vi "DSF.Engine.Interface.Transceiver.Write.Command.vi"(6 "overwrite on timeout (T)":bool, 8 "error in (no error)":errorcluster, 9 "timeout in ms (0)":i32 format="%d ms", 10 "command":T1, 11 "Transceiver Interface in":refnum<class "DSF.Engine.Interface.Transceiver.lvclass">) -> (0 "error out":errorcluster, 1 "timed out?":bool, 3 "Transceiver Interface out":refnum<class "DSF.Engine.Interface.Transceiver.lvclass">)   [LabVIEW 2017, in "DSF.Engine.lvlib" / "DSF.Engine.Interface.Transceiver.lvclass"]
uses:
  DSF.Engine.Interface.Transceiver.lvclass
  C:/Git/DSF/Source/Engine/Classes/Interface/DSF.Engine.Interface.lvclass
  DSF.Engine.Interface.Transceiver.Command Data.ctl
  DSF.Engine.Interface.Transceiver.Command.ctl
  DSF.Engine.Interface.Transceiver.Command Parameters.ctl
  DSF.Engine.Interface.RT FIFO.Data.16B.ctl
  DSF.Engine.Interface.RT FIFO.Payload.16B.ctl
  DSF.Engine.Interface.lvclass/DSF.Engine.Interface.ctl
  Debug/DSF.Engine.Debug Flags.FIFO.lvclass/DSF.Engine.Debug Flags.FIFO.ctl
  DSF.Engine.Interface.Get Command FIFO.vi
  DSF.Engine.Interface.RT FIFO.Write.16B.vi
  DSF.Engine.Interface.Get Debug Flags.vi
  Debug/DSF.Engine.Debug Flags.FIFO.Get Infinite Timeouts.vi
  DSF.Engine.Interface.lvclass
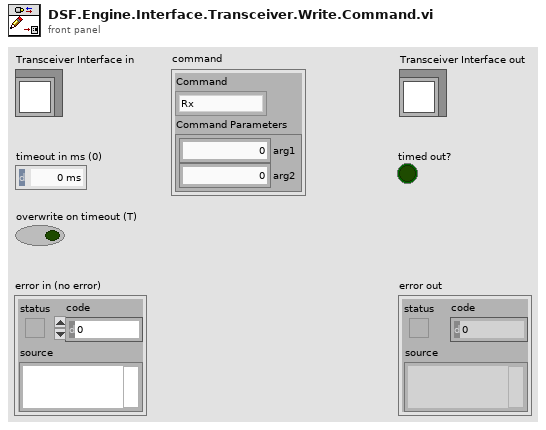
[diagram p1: front panel]
types:
  T1 = typedef "DSF.Engine.lvlib/DSF.Engine.Interface.Transceiver.lvclass/DSF.Engine.Interface.Transceiver.Command Data.ctl" = cluster{"Command":T2, "Command Parameters":T3}
  T2 = typedef "DSF.Engine.lvlib/DSF.Engine.Interface.Transceiver.lvclass/DSF.Engine.Interface.Transceiver.Command.ctl" = enum8{"Rx", "Tx", "Shutdown"}
  T3 = typedef "DSF.Engine.lvlib/DSF.Engine.Interface.Transceiver.lvclass/DSF.Engine.Interface.Transceiver.Command Parameters.ctl" = cluster{"arg1":u64, "arg2":u64}
  T4 = typedef "DSF.Engine.lvlib/DSF.Engine.Interface.lvclass/DSF.Engine.Interface.RT FIFO.Data.16B.ctl" = cluster{"Command":u8, "Payload":T5}
  T5 = typedef "DSF.Engine.lvlib/DSF.Engine.Interface.lvclass/DSF.Engine.Interface.RT FIFO.Payload.16B.ctl" = cluster{"arg1":u64, "arg2":u64}
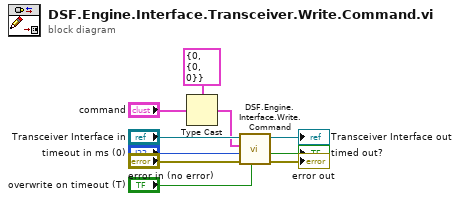
[diagram p0: block diagram]
diagram:
  n1 = Type Cast(type=T4 {"Command"=0, "Payload"={"arg1"=0, "arg2"=0}} ("element"), x="command") -> (*(type *) &x=w7:T4)
  n2 = call "DSF.Engine.Interface.Write.Command.vi"("overwrite on timeout (T)"="overwrite on timeout (T)", "error in (no error)"="error in (no error)", "timeout in ms (0)"="timeout in ms (0)", "command"=w7, "Interface in"="Transceiver Interface in") -> ("error out"=→"error out":errorcluster, "timed out?"=→"timed out?":bool, "Interface out"=→"Transceiver Interface out":refnum<class "DSF.Engine.Interface.Transceiver.lvclass">)  [unwired: 4 in]
